vi "Send Config Command.vi"(9 "Config Command":string="AT*CONFIG=1,\"general:navdata_demo\",\"TRUE\"", 10 "NavData Port":refnum<k16>, 11 "AT Command Port":refnum<k16>) -> (2 "NavData Port":refnum<k16>, 3 "AT Command Port":refnum<k16>)   [LabVIEW 2011]
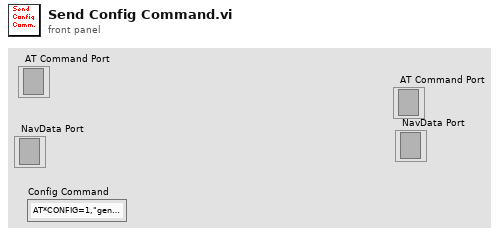
[diagram p1: front panel]
types:
  T1 = cluster{"Drone Status Bits":cluster{"Flying?":bool, "Video Enabled?":bool, "Vision Enabled?":bool, "Angular Speed Control?":bool, "Altitude Control?":bool, "Start button?":bool, "Control Command Recieved?":bool, "Trim Command Recieved?":bool, "Trim Running?":bool, "Trim Succeeded?":bool, "Navdata Demo Mode?":bool, "Navdata Bootstrap Mode?":bool, "Motors Com Down?":bool, "Unknown":bool, "Gyrometer Problem?":bool, "Battery Voltage Too Low?":bool, "Battery Voltage Too High?":bool, "Timer Elapsed?":bool, "Power Too Low?":bool, "Angles Out Of Range?":bool, "Too Much Wind?":bool, "Ultrasound Deaf?":bool, "Cutout Detected?":bool, "PIC Version Number OK?":bool, "ATCodec Thread On?":bool, "Navdata Thread On?":bool, "Video Thread On?":bool, "Acquisition Thread On?":bool, "Control Watchdog Delay?":bool, "ADC Watchdog Delay?":bool, "Communications Problem?":bool, "Emergency?":bool}, "Header":u32, "Sequence Number":u32, "Vision Defined?":bool, "Blocks":cluster{"Size":u16, "Data":u8[], "ID":enum16{"NAVDATA_DEMO", "NAVDATA_TIME", "NAVDATA_RAW_MEASURES", "NAVDATA_PHYS_MEASURES", "NAVDATA_GYROS_OFFSETS", "NAVDATA_EULER_ANGLES", "NAVDATA_REFERENCES", "NAVDATA_TRIMS", "NAVDATA_RC_REFERENCES", "NAVDATA_PWM", "NAVDATA_ALTITUDE", "NAVDATA_VISION_RAW", "NAVDATA_VISION_OF", "NAVDATA_VISION", "NAVDATA_VISION_PERF", "NAVDATA_TRACKERS_SEND", "NAVDATA_VISION_DETECT", "NAVDATA_WATCHDOG", "NAVDATA_ADC_DATA_FRAME", "NAVDATA_VIDEO_STREAM", "NAVDATA_GAMES"}}[]}
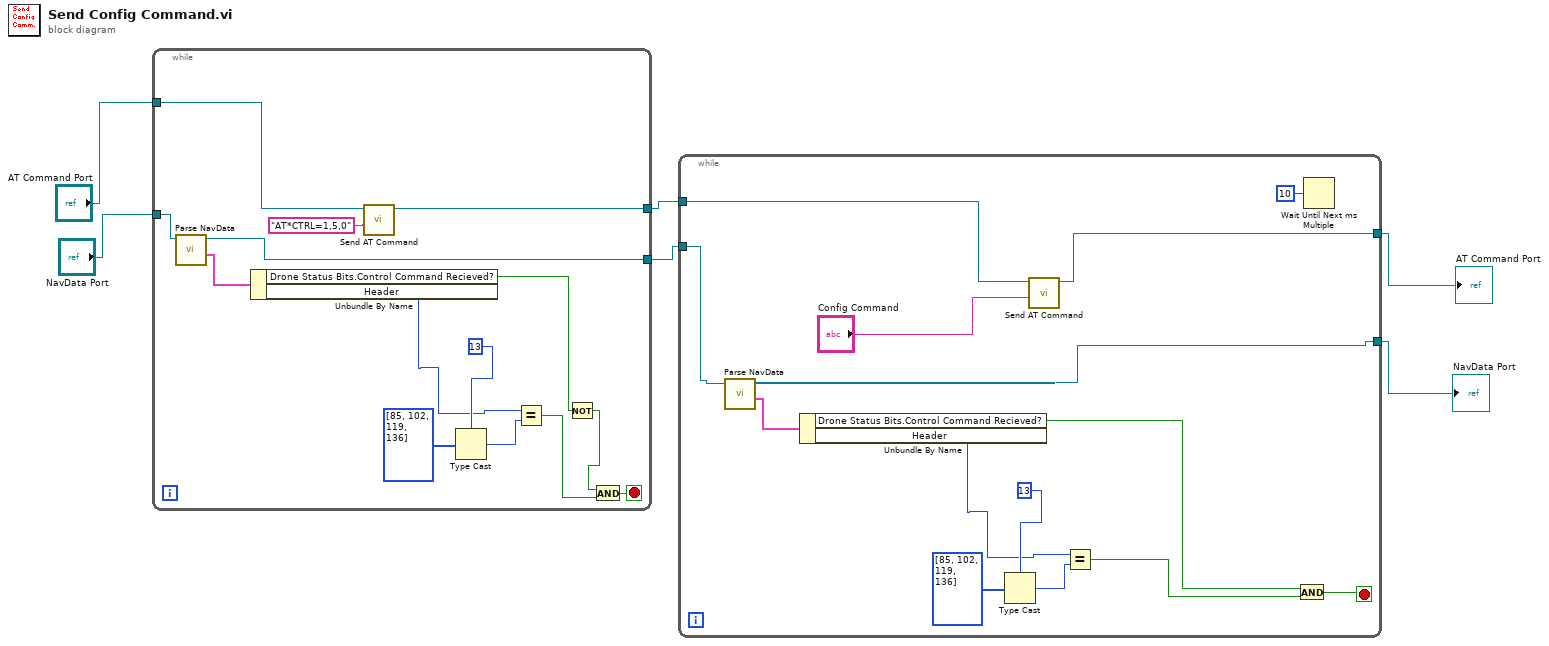
[diagram p0: block diagram]
diagram:
  n1 = while {
    tunnel: "AT Command Port" -> [w19]
    tunnel: "NavData Port" -> [w13]
    tunnel: [w10] -> w5
    tunnel: [w9] -> w6
    stop <- w12 stop-if-true
    n2 = call "Parse NavData.vi"("NavData Port"=w13) -> ("NavData"=w15:T1, "NavData Port"=w10:refnum<k16>)  [unwired: 9 in]
    n3 = Unbundle By Name(w15) -> ("Drone Status Bits.Control Command Recieved?"=w7:bool, "Header"=w14:u32)
    n4 = call "Send AT Command.vi"("AT Command"="AT*CTRL=1,5,0", "AT Command Port"=w19) -> ("AT Command Port"=w9:refnum<k16>)  [unwired: 9 in]
    n5 = Type Cast(type=u32 13, x=u8[] [85, 102, 119, 136]) -> (*(type *) &x=w16:u32)
    n6 = Equal?(x=w14, y=w16) -> (x = y?=w11:bool)
    n7 = Not(x=w7) -> (.not. x?=w8:bool)
    n8 = And(x=w8, y=w11) -> (x .and. y?=w12:bool)
  }
  n9 = while {
    tunnel: w6 -> [w29]
    tunnel: [w27] -> w1
    tunnel: w5 -> [w28]
    tunnel: [w26] -> w2
    stop <- w23 stop-if-true
    n10 = call "Parse NavData.vi"("NavData Port"=w28) -> ("NavData"=w25:T1, "NavData Port"=w27:refnum<k16>)  [unwired: 9 in]
    n11 = Unbundle By Name(w25) -> ("Drone Status Bits.Control Command Recieved?"=w22:bool, "Header"=w24:u32)
    n12 = Type Cast(type=u32 13, x=u8[] [85, 102, 119, 136]) -> (*(type *) &x=w31:u32)
    n13 = call "Send AT Command.vi"("AT Command"="Config Command", "AT Command Port"=w29) -> ("AT Command Port"=w26:refnum<k16>)  [unwired: 9 in]
    n14 = Equal?(x=w24, y=w31) -> (x = y?=w21:bool)
    n15 = And(x=w22, y=w21) -> (x .and. y?=w23:bool)
    n16 = Wait Until Next ms Multiple(millisecond multiple=u32 10) -> ()  [unwired: 1 out]
  }
  "AT Command Port" <- w2
  "NavData Port" <- w1
